vi "Limit Test.vi"(8 "error in (no error)":errorcluster, 9 "Filter Error Limits":dbl, 10 "Number of Steps":i32=25, 11 "Freq Amp Array":dbl[][](array[numeric])) -> (0 "error out":errorcluster, 2 "Limit Test Results":cluster{dbl[], dbl[]}[](graph)=[{[1000.0, 9166.666666666668, 17333.333333333336, 25500.0, 33666.66666666667, 41833.333333333336, 50000.0], [0.8109999999999999, 0.7375, 0.6639999999999999, 0.5905, 0.5169999999999999, 0.44349999999999995, 0.37]}, {[1000.0, 9166.666666666668, 17333.333333333336, 25500.0, 33666.66666666667, 41833.333333333336, 50000.0], [0.7727256581908878, 0.7031032017391705, 0.5983315439720234, 0.5084307021460196, 0.4381322995151595, 0.3914920131543004, 0.35634281183887034]}, {[1000.0, 9166.666666666668, 17333.333333333336, 25500.0, 33666.66666666667, 41833.333333333336, 50000.0], [0.6910000000000001, 0.6174999999999999, 0.544, 0.4705, 0.39699999999999996, 0.32349999999999995, 0.25]}], 3 "Test Passed?":bool)   [LabVIEW 2010]
doc: "Takes the raw data from the <b>FreqSweepTest VI</b> and filter error limits and then calculates if the filter response data ever went out of bounds. If they did not, then the limit test passed and the VI outputs a \"True\" from the \"Test Passed\" indicator. It also outputs a waveform graph showing the results of the frequency sweep test and the limits."
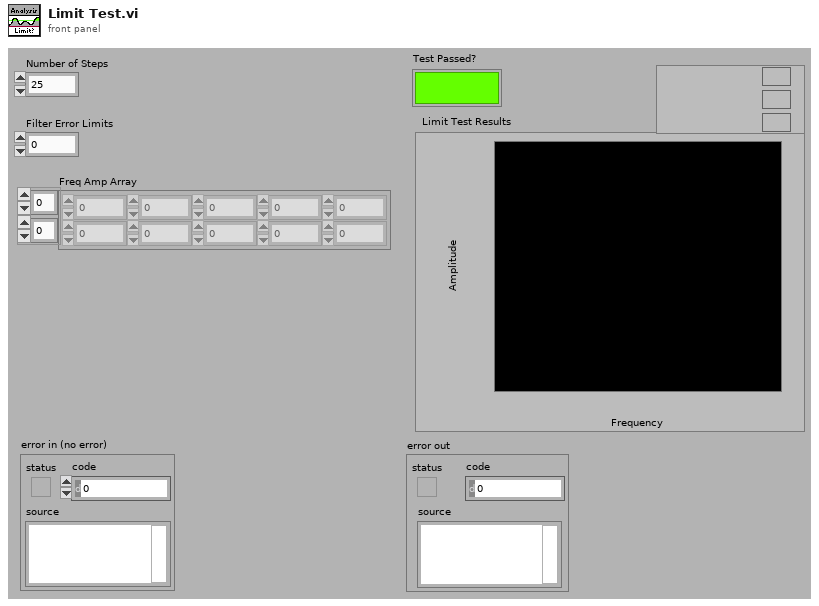
[diagram p1: front panel]
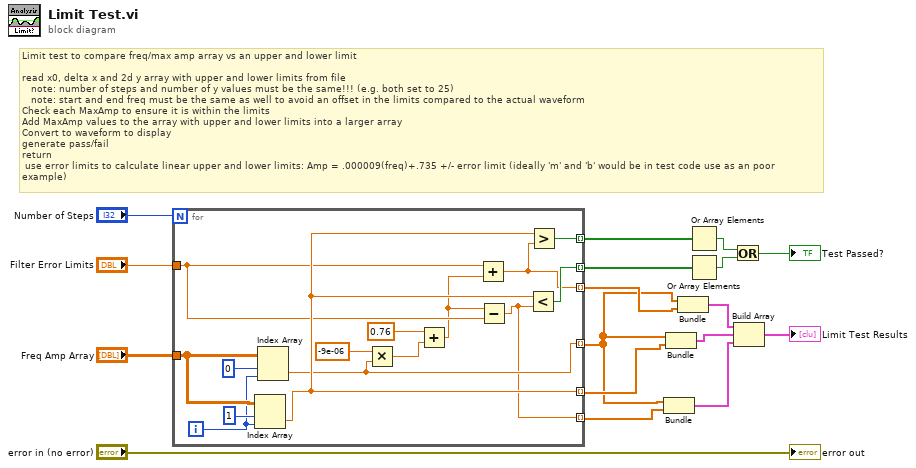
[diagram p0: block diagram]
diagram:
  # "Limit test to compare freq/max amp array vs an upper and lower limit\n\nread x0, delta x and 2d y array with upper and lower limits from file\n   note: number of steps and number of y values must be the same!!! (e.g. both set to 25)\n   note: start and end freq must be the same as well to avoid an offset in the limits compared to the actual waveform\nCheck each MaxAmp to ensure it is within the limits\nAdd MaxAmp values to the array with upper and lower limits into a larger array\nConvert to waveform to display\ngenerate pass/fail\nreturn\n use error limits to calculate linear upper and lower limits: Amp = .000009(freq)+.735 +/- error limit (ideally 'm' and 'b' would be in test code use as an poor example)"
  n1 = for {
    N: "Number of Steps" -> [_]
    tunnel: "Freq Amp Array" -> [w28]
    tunnel: [w26] -> w10 mode=indexing
    tunnel: [w21] -> w11 mode=indexing
    tunnel: [w31] -> w16 mode=indexing
    tunnel: [w30] -> w15 mode=indexing
    tunnel: [w18] -> w8 mode=indexing
    tunnel: [w22] -> w9 mode=indexing
    tunnel: "Filter Error Limits" -> [w20]
    i -> [w27]
    n2 = Index Array(array=w28, index (row)=1 ("index"), index (col)=w27) -> (element=w26:dbl)
    n3 = Index Array(array=w28, index (row)=0 ("index"), index (col)=w27) -> (element=w22:dbl)
    n4 = Multiply(x=-9e-06 ("element"), y=w22) -> (x*y=w24:dbl)
    n5 = Add(x=0.76 ("element"), y=w24) -> (x+y=w19:dbl)
    n6 = Add(x=w20, y=w19) -> (x+y=w21:dbl)
    n7 = Subtract(x=w19, y=w20) -> (x-y=w18:dbl)
    n8 = Less?(x=w26, y=w18) -> (x < y?=w30:bool)
    n9 = Greater?(x=w26, y=w21) -> (0:w31:bool)
  }
  n10 = Bundle(w9, w8) -> (w5:cluster{dbl[], dbl[]})  [unwired: 1 out]
  n11 = Bundle(w9, w10) -> (w6:cluster{dbl[], dbl[]})  [unwired: 1 out]
  n12 = Bundle(w9, w11) -> (w7:cluster{dbl[], dbl[]})  [unwired: 1 out]
  n13 = Or Array Elements(Boolean array=w16) -> (logical OR=w14:bool)
  n14 = Or Array Elements(Boolean array=w15) -> (logical OR=w13:bool)
  n15 = Or(x=w14, y=w13) -> (x .or. y?=→"Test Passed?":bool)
  n16 = Build Array "Build Array"(w7, w6, w5) -> (→"Limit Test Results":cluster{dbl[], dbl[]}[])
  "error out" <- "error in (no error)"
